vi "Fibonacci.vi"() -> ()   [LabVIEW 2018]
panel:
  out "output":dbl
  in  "Boolean":bool
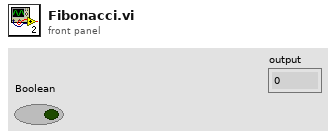
[diagram p1: front panel]
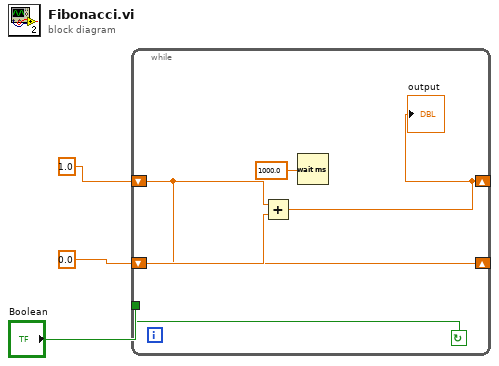
[diagram p0: block diagram]
diagram:
  n1 = while {
    tunnel: "Boolean" -> [w8]
    shift-right: [w6] -> _
    shift-left: 1.0 ("Numeric") -> [w5]
    shift-right: [w5] -> _
    shift-left: 0.0 ("Numeric") -> [w7]
    stop <- w8 continue-if-true
    n2 = Add(x=w5, y=w7) -> (x+y=w6:dbl)
    "output" <- w6
    n3 = Wait (ms)(milliseconds to wait=1000.0 ("Numeric")) -> ()  [unwired: 1 out]
  }
